vi "Begin.vi"(8 "error in":errorcluster) -> (0 "error out":errorcluster)   [LabVIEW 2018]
doc: "Called before other user functions, this VI is expected to open initial I/O refnums, load in file data, and do all program initialization. Notice that the <B>error out</B> terminal is simply used for data flow. Wiring it to other structures or subVIs ensures that this VI runs first."
uses:
  <vilib>/Rock Robotics/SystemInterfaces/DIO/FPGA_DIOPWMChannel.ctl
  <vilib>/Rock Robotics/WPI/SafetyOutput/WPI_SafetyOutputConfigMenu.ctl
  <vilib>/Rock Robotics/WPI/DriverStation/WPI_DriverStationRobotMode2.ctl
  <vilib>/Rock Robotics/WPI/Joystick/WPI_JoystickDeviceEnum.ctl
  <vilib>/Rock Robotics/WPI/Solenoid/WPI_SolenoidChannel.ctl
  <vilib>/Rock Robotics/SystemInterfaces/spilib/spi_bus.ctl
  Robot Global Data.vi
  <vilib>/Rock Robotics/Network Tables/NT Write String Array.vi
  <vilib>/Rock Robotics/WPI/RobotDrive/WPI_RobotDriveOpen4MotorWithSPARK.vi
  <vilib>/Rock Robotics/WPI/Utilities/WPI_GetSetVariantRefNum.vi
  <vilib>/Rock Robotics/WPI/Solenoid/WPI_SolenoidOpenDouble.vi
  <vilib>/Rock Robotics/WPI/MotorControl/WPI_MotorControlOpen SPARK.vi
  <vilib>/Rock Robotics/WPI/Gyro/WPI_GyroXRS450_SPI_Open.vi
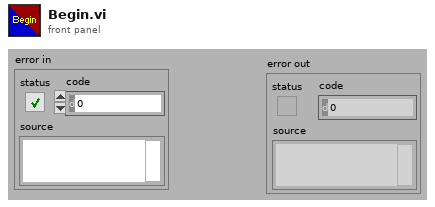
[diagram p1: front panel]
types:
  T1 = typedef "spi_bus.ctl" = enum16{"SPI On-Board, CS0", "SPI On-Board, CS1", "SPI On-Board, CS2", "SPI On-Board, CS3", "SPI MXP", "Invalid"}
  T2 = typedef "FPGA_DIOPWMChannel.ctl" = enum8{"PWM 0", "PWM 1", "PWM 2", "PWM 3", "PWM 4", "PWM 5", "PWM 6", "PWM 7", "PWM 8", "PWM 9", "PWM MXP 0", "PWM MXP 1", "PWM MXP 2", "PWM MXP 3", "PWM MXP 4", "PWM MXP 5", "PWM MXP 6", "PWM MXP 7", "PWM MXP 8", "PWM MXP 9", "Invalid"}
  T3 = typedef "WPI_SolenoidChannel.ctl" = enum8{"Solenoid 0", "Solenoid 1", "Solenoid 2", "Solenoid 3", "Solenoid 4", "Solenoid 5", "Solenoid 6", "Solenoid 7", "Invalid"}
  T4 = typedef "WPI_JoystickDeviceEnum.ctl" = enum16{"USB 0", "USB 1", "USB 2", "USB 3", "USB 4", "USB 5"}
  T5 = typedef "WPI_DriverStationRobotMode2.ctl" = enum16{"Autonomous Disabled", "Autonomous Enabled", "Teleop Disabled", "Teleop Enabled", "Disconnected", "Finish", "Test Disabled", "Test Enabled", "Emergency Stopped"}
  T6 = typedef "WPI_SafetyOutputConfigMenu.ctl" = enum16{"Enable", "Disable"}
  T7 = typedef "WPI_CompressorDevRef.ctl" = cluster{"DevStatus":errorcluster, "Pneumatics Control Module":u8}
  T8 = typedef "WPI_MotorControlDeviceRef.ctl" = cluster{"DeviceStatus":errorcluster, "Type":T9, "PWM":cluster{"PWM Channel":T2, "DeadBand":T10}, "CAN":cluster{"Device Number":u8, "SetOutput VI Ref":variant, "GetOutput VI Ref":variant, "Enable VI Ref":variant, "Disable VI Ref":variant, "Data":variant}, "Invert":bool, "DIO PWM":cluster{"PWM \"Enable\" Channel":T2, "DIOChannel":T11, "PWM Rate":dbl}}
  T9 = typedef "WPI_MotorControlType.ctl" = enum16{"PWM", "CAN", "DIO PWM"}
  T10 = typedef "WPI_PWMDeadband.ctl" = cluster{"Name":string, "maxPositivePwm":i32, "minPositivePwm":i32, "centerPwm":i32, "maxNegativePwm":i32, "minNegativePwm":i32, "angularRange":u16}
  T11 = typedef "FPGA_DIOChannel.ctl" = enum8{"DIO 0", "DIO 1", "DIO 2", "DIO 3", "DIO 4", "DIO 5", "DIO 6", "DIO 7", "DIO 8", "DIO 9", "DIO MXP 0", "DIO MXP 1", "DIO MXP 2", "DIO MXP 3", "DIO MXP 4", "DIO MXP 5", "DIO MXP 6", "DIO MXP 7", "DIO MXP 8", "DIO MXP 9", "DIO MXP 10", "DIO MXP 11", "DIO MXP 12", "DIO MXP 13", "DIO MXP 14", "DIO MXP 15", "SPI Port CS1", "SPI Port CS2", "SPI Port CS3", "SPI Port MISO", "SPI Port MOSI", "Invalid"}
  T12 = typedef "WPI_JoystickDevRef.ctl" = cluster{"Device":T4}
  T13 = typedef "WPI_SolenoidDevRef.ctl" = cluster{"DevStatus":errorcluster, "Pneumatics Control Module":u8, "Forward Solenoid Channel":T3, "Reverse Solenoid Channel":T3}
  T14 = typedef "WPI_RobotDriveDevRef.ctl" = cluster{"DevStatus":errorcluster, "Motors[]":T8[], "Square Inputs":bool, "Max Output":dbl}
  T15 = typedef "WPI_GyroDevRef.ctl" = cluster{"DevStatus":errorcluster, "Analog Channel":T16, "Gain (VoltsPerDegree/Second)":dbl, "Gyro Type":enum16{"Analog", "XRS450"}, "Handle":i32, "SPI Bus":T1, "Device Found":bool, "Sample Rate":dbl, "Calibrate On Open":bool, "Offset":dbl}
  T16 = typedef "FPGA_AIChannel.ctl" = enum8{"AI 0", "AI 1", "AI 2", "AI 3", "AI MXP 0", "AI MXP 1", "AI MXP 2", "AI MXP 3", "Invalid"}
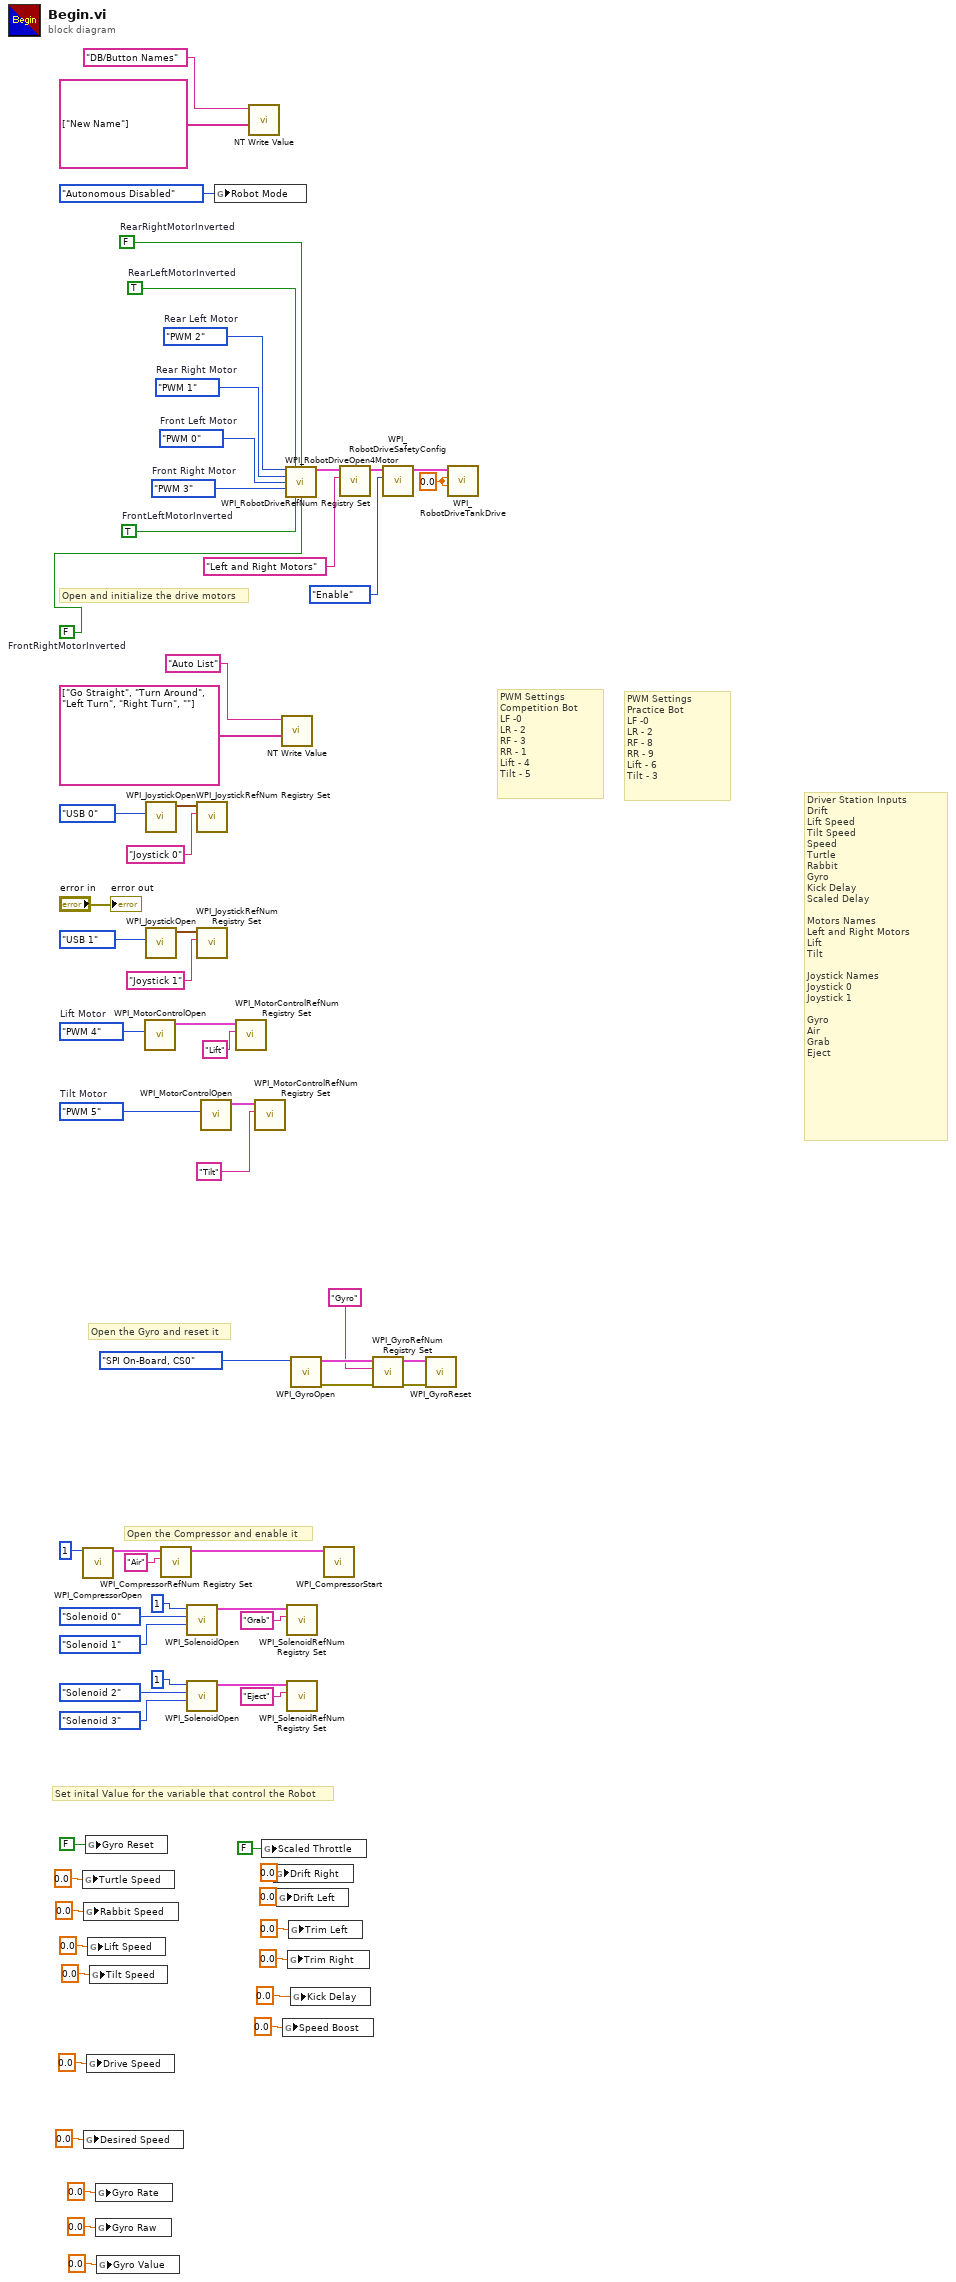
[diagram p0: block diagram]
diagram:
  w11 = FPGA_DIOPWMChannel."PWM 5"  # Tilt Motor
  w14 = FPGA_DIOPWMChannel."PWM 4"  # Lift Motor
  w26 = 0.0 ("Left axis value")
  w49 = FALSE  # FrontRightMotorInverted
  w50 = TRUE  # FrontLeftMotorInverted
  w53 = FPGA_DIOPWMChannel."PWM 3"  # Front Right Motor
  w54 = FPGA_DIOPWMChannel."PWM 0"  # Front Left Motor
  w55 = FPGA_DIOPWMChannel."PWM 1"  # Rear Right Motor
  w56 = FPGA_DIOPWMChannel."PWM 2"  # Rear Left Motor
  w51 = TRUE  # RearLeftMotorInverted
  w52 = FALSE  # RearRightMotorInverted
  # "PWM Settings \nPractice Bot\nLF -0\nLR - 2\nRF - 8\nRR - 9\nLift - 6\nTilt - 3"
  # "PWM Settings \nCompetition Bot\nLF -0\nLR - 2\nRF - 3\nRR - 1\nLift - 4\nTilt - 5"
  # "Driver Station Inputs\nDrift\nLift Speed\nTilt Speed\nSpeed\nTurtle\nRabbit\nGyro\nKick Delay\nScaled Delay\n\nMotors Names\nLeft and Right Motors\nLift\nTilt\n\nJoystick Names\nJoystick 0\nJoystick 1\n\nGyro\nAir\nGrab\nEject"
  # "Open the Gyro and reset it"
  # "Set inital Value for the variable that control the Robot"
  # "Open and initialize the drive motors"
  # "Open the Compressor and enable it"
  n1 = call <vilib>:"WPI_CompressorOpen.vi"("Pneumatics Control Module (0)"=u8 1) -> ("CompressorDevRef"=w45:T7)  [unwired: 13 in, 1 out]
  n2 = global write "Robot Global Data.vi" "Turtle Speed"(0.0 ("Alliance")) -> ()
  n3 = global write "Robot Global Data.vi" "Rabbit Speed"(0.0 ("Alliance")) -> ()
  n4 = global write "Robot Global Data.vi" "Desired Speed"(0.0 ("Alliance")) -> ()
  n5 = global write "Robot Global Data.vi" "Gyro Reset"(FALSE ("Gyro Reset")) -> ()
  n6 = global write "Robot Global Data.vi" "Drive Speed"(0.0 ("Alliance")) -> ()
  n7 = global write "Robot Global Data.vi" "Lift Speed"(0.0 ("Alliance")) -> ()
  n8 = global write "Robot Global Data.vi" "Tilt Speed"(0.0 ("Alliance")) -> ()
  n9 = global write "Robot Global Data.vi" "Gyro Rate"(0.0 ("Alliance")) -> ()
  n10 = global write "Robot Global Data.vi" "Gyro Raw"(0.0 ("Alliance")) -> ()
  n11 = global write "Robot Global Data.vi" "Gyro Value"(0.0 ("Alliance")) -> ()
  n12 = call-poly <vilib>:"WPI_MotorControlOpen.vi"("PWM Channel"=w14) -> ("MotorControlDeviceRef"=w16:T8)  [unwired: 9 in, 1 out]
  n13 = call <vilib>:"WPI_JoystickOpen.vi"("JoystickDevice"=WPI_JoystickDeviceEnum."USB 0") -> ("JoystickDevRef"=w64:T12)  [unwired: 10 in]
  n14 = call <vilib>:"WPI_JoystickOpen.vi"("JoystickDevice"=WPI_JoystickDeviceEnum."USB 1") -> ("JoystickDevRef"=w47:T12)  [unwired: 10 in]
  n15 = call <vilib>:"WPI_CompressorRefNum Registry Set.vi"("refnum name"="Air", "CompressorDevRef"=w45) -> ("CompressorDevRef"=w43:T7)  [unwired: 8 in, 1 out]
  n16 = call-poly <vilib>:"WPI_SolenoidOpen.vi"("Reverse Solenoid Channel"=WPI_SolenoidChannel."Solenoid 1", "Forward Solenoid Channel"=WPI_SolenoidChannel."Solenoid 0", "Pneumatics Control Module (0)"=u8 1) -> ("SolenoidDevRef"=w32:T13)  [unwired: 7 in, 1 out]
  n17 = call-poly <vilib>:"WPI_SolenoidOpen.vi"("Reverse Solenoid Channel"=WPI_SolenoidChannel."Solenoid 3", "Forward Solenoid Channel"=WPI_SolenoidChannel."Solenoid 2", "Pneumatics Control Module (0)"=u8 1) -> ("SolenoidDevRef"=w37:T13)  [unwired: 7 in, 1 out]
  n18 = call <vilib>:"WPI_JoystickRefNum Registry Set.vi"("refnum name"="Joystick 0", "JoystickDevRef"=w64) -> ()  [unwired: 8 in, 2 out]
  n19 = call <vilib>:"WPI_JoystickRefNum Registry Set.vi"("refnum name"="Joystick 1", "JoystickDevRef"=w47) -> ()  [unwired: 8 in, 2 out]
  n20 = call-poly <vilib>:"WPI_MotorControlOpen.vi"("PWM Channel"=w11) -> ("MotorControlDeviceRef"=w13:T8)  [unwired: 9 in, 1 out]
  n21 = global write "Robot Global Data.vi" "Robot Mode"(WPI_DriverStationRobotMode2."Autonomous Disabled" ("Robot Mode")) -> ()
  n22 = call <vilib>:"WPI_MotorControlRefNum Registry Set.vi"("refnum name"="Lift", "MotorControlDevRef"=w16) -> ()  [unwired: 8 in, 2 out]
  n23 = call-poly <vilib>:"NT Write Value.vi"("String Array"=string[] ["New Name"], "Name"="DB/Button Names") -> ()  [unwired: 9 in, 1 out]
  n24 = call <vilib>:"WPI_MotorControlRefNum Registry Set.vi"("refnum name"="Tilt", "MotorControlDevRef"=w13) -> ()  [unwired: 8 in, 2 out]
  n25 = global write "Robot Global Data.vi" "Scaled Throttle"(FALSE ("Scaled Throttle")) -> ()
  n26 = global write "Robot Global Data.vi" "Drift Right"(0.0 ("Drift")) -> ()
  n27 = global write "Robot Global Data.vi" "Drift Left"(0.0 ("Drift")) -> ()
  n28 = call-poly <vilib>:"NT Write Value.vi"("String Array"=string[] ["Go Straight", "Turn Around", "Left Turn", "Right Turn", ""], "Name"="Auto List") -> ()  [unwired: 9 in, 1 out]
  n29 = global write "Robot Global Data.vi" "Speed Boost"(0.0 ("Alliance")) -> ()
  n30 = call-poly <vilib>:"WPI_RobotDriveOpen4Motor.vi"("Rear Left Motor"=w56, "Rear Left Motor Inverted"=w51, "Rear Right Motor Inverted"=w52, "Rear Right Motor"=w55, "Front Left Motor"=w54, "Front Right Motor"=w53, "Front Left Motor Inverted"=w50, "Front Right Motor Inverted"=w49) -> ("RobotDriveDevRef"=w57:T14)  [unwired: 6 in, 1 out]
  n31 = call <vilib>:"WPI_SolenoidRefNum Registry Set.vi"("refnum name"="Grab", "SolenoidDevRef"=w32) -> ()  [unwired: 8 in, 2 out]
  n32 = call <vilib>:"WPI_SolenoidRefNum Registry Set.vi"("refnum name"="Eject", "SolenoidDevRef"=w37) -> ()  [unwired: 8 in, 2 out]
  n33 = global write "Robot Global Data.vi" "Trim Right"(0.0 ("Alliance")) -> ()
  n34 = global write "Robot Global Data.vi" "Trim Left"(0.0 ("Alliance")) -> ()
  n35 = call-poly <vilib>:"WPI_GyroOpen.vi"("SPI Bus"=spi_bus."SPI On-Board, CS0") -> ("error out"=w6:errorcluster, "GyroDevRef"=w7:T15)  [unwired: 8 in, 1 out]
  n36 = global write "Robot Global Data.vi" "Kick Delay"(0.0 ("Alliance")) -> ()
  n37 = call <vilib>:"WPI_CompressorStart.vi"("CompressorDevRef"=w43) -> ()  [unwired: 9 in, 2 out]
  n38 = call <vilib>:"WPI_RobotDriveRefNum Registry Set.vi"("refnum name"="Left and Right Motors", "RobotDriveDevRef"=w57) -> ("RobotDriveDevRef"=w68:T14)  [unwired: 2 in, 7 out]
  n39 = call <vilib>:"WPI_GyroRefNum Registry Set.vi"("error in (no error)"=w6, "refnum name"="Gyro", "GyroDevRef"=w7) -> ("error out"=w10:errorcluster, "GyroDevRef"=w9:T15)  [unwired: 7 in]
  n40 = call <vilib>:"WPI_RobotDriveSafetyConfig.vi"("mode"=WPI_SafetyOutputConfigMenu."Enable", "RobotDriveDevRef"=w68) -> ("RobotDriveDevRef"=w27:T14)  [unwired: 8 in, 1 out]
  n41 = call <vilib>:"WPI_GyroReset.vi"("error in"=w10, "GyroDevRef"=w9) -> ()  [unwired: 8 in, 2 out]
  n42 = call <vilib>:"WPI_RobotDriveTankDrive.vi"("Right axis value"=w26, "Left axis value"=w26, "RobotDriveDevRef"=w27) -> ()  [unwired: 6 in, 3 out]
  "error out" <- "error in"
